vi "Load Cfg.vi"(8 "error in (no error)":errorcluster, 11 "Communication Channel in":refnum<class "Communication Channel.lvclass">) -> (0 "error out":errorcluster, 3 "Communication Channel out":refnum<class "Communication Channel.lvclass">)   [LabVIEW 2018, in "Communication Channel.lvclass"]
uses:
  Communication Channel.lvclass
  <vilib>/Utility/config.llb/NI_LVConfig.lvlib
  <vilib>/Utility/config.llb/Read Key (String).vi
  Socket/Socket.lvclass
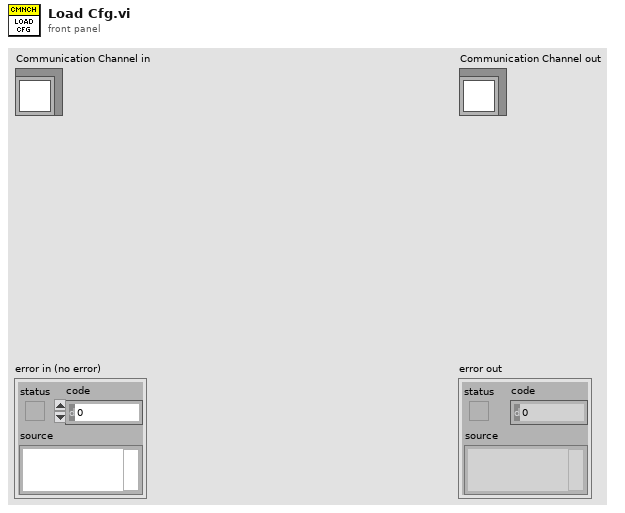
[diagram p1: front panel]
types:
  T1 = typedef "NI_LVConfig.lvlib/Config Data RefNum.ctl" = refnum<k1>
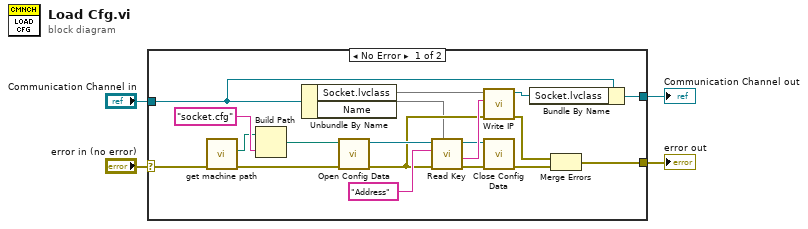
[diagram p0: block diagram]
diagram:
  n1 = case shown="No Error" "error in (no error)" {
    selector: "error in (no error)" -> [w10 w25]
    tunnel: [w13 w25] -> w3
    tunnel: [w15 w24] -> w1
    tunnel: "Communication Channel in" -> [w16 w24]
    frame No Error {
      n2 = call "get machine path.vi"("error in (no error) 2"=w10) -> ("error in (no error)"=w9:errorcluster, "machine path"=w11:path)  [unwired: 9 in]
      n3 = Build Path(base path=w11, name or relative path="socket.cfg") -> (appended path=w23:path)
      n4 = Unbundle By Name(w16) -> ("Socket.lvclass"=w5, "Name"=w8)
      n5 = call <vilib>:"Open Config Data.vi"("error in (no error)"=w9, "configuration file path"=w23) -> ("error out"=w12:errorcluster, "refnum"=w20:T1)  [unwired: 7 in, 1 out]
      n6 = call-poly <vilib>:"Read Key.vi"("section"=w8, "error in (no error)"=w12, "key"="Address", "refnum"=w20) -> ("error out"=w6:errorcluster, "value"=w19:string, "refnum out"=w7:T1)  [unwired: 4 in, 1 out]
      n7 = call-dynamic "Write IP.vi"("error in (no error)"=w12, "IP"=w19, "Socket in"=w5) -> ("error out"=w18:errorcluster, "Socket out"=w17:refnum<class "Socket.lvclass">)  [unwired: 7 in]
      n8 = call <vilib>:"Close Config Data.vi"("error in (no error)"=w6, "refnum"=w7) -> ("error out"=w14:errorcluster)  [unwired: 8 in, 1 out]
      n9 = Bundle By Name(cluster=w16, "Socket.lvclass"=w17) -> (w15:refnum<class "Communication Channel.lvclass">)
      n10 = Merge Errors(w18, w14) -> (w13:errorcluster)
    }
    frame Error {
    }
  }
  "error out" <- w3
  "Communication Channel out" <- w1
